vi "rem_killOcc.vi"(0 "Host_Reference":refnum<class "HGF_Reference.lvclass">, 2 "timeout in ms (-1)":i32, 3 "ID":string, 5 "error in (no error)":errorcluster) -> (14 "dup Host_Reference":refnum<class "HGF_Reference.lvclass">, 16 "dup timeout in ms (-1)":i32, 19 "error out":errorcluster)   [LabVIEW 2009, in "MoAgSy.lvlib" / "MoAgSy_Host.lvclass"]
doc: "<B>public</B> VI removes kill occurence from referenced Host.\nOccurrence is specified by the Agents ID.\n\nF.Berck@gsi.de\nGSI Darmstadt 2009"
uses:
  MoAgSy_Host.lvclass
  HGF_BaseClasses/HGF_Reference/HGF_Reference.lvclass
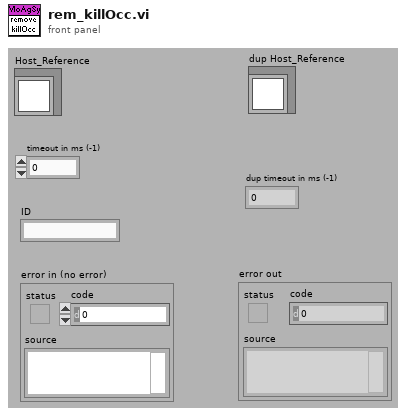
[diagram p1: front panel]
types:
  T1 = cluster{"killNotifier":refnum<notifier>, "Agent ID":string}[]
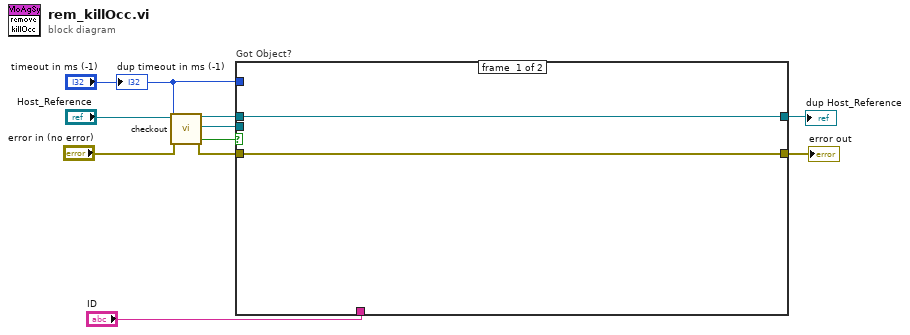
[diagram p0: block diagram]
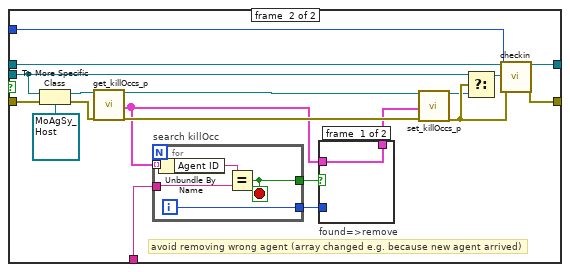
[diagram p2: hidden frame]
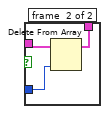
[diagram p3: hidden frame]
diagram:
  n1 = call "checkout.vi"("HGF_Reference"="Host_Reference", "timeout in ms (-1)"="timeout in ms (-1)", "error in (no error)"="error in (no error)") -> ("dup HGF_Reference"=w5:refnum<class "HGF_Reference.lvclass">, "Object"=w3:refnum<class>, "got object?"=w4:bool, "error out"=w2:errorcluster)  [unwired: 13 out]
  n2 = case "Got Object?" shown="True" w4 {
    tunnel: w3 -> [_ w25]
    tunnel: w5 -> [w12 w30]
    tunnel: [w12 w29] -> w8
    tunnel: "timeout in ms (-1)" -> [_ w28]
    tunnel: [w11 w27] -> w9
    tunnel: w2 -> [w11 w26]
    tunnel: "ID" -> [_ w17]
    frame #0 {
    }
    frame #1 {
      # "avoid removing wrong agent (array changed e.g. because new agent arrived)"
      n3 = To More Specific Class(target class=refnum<class "MoAgSy_Host.lvclass"> refnum ("MoAgSy.lvlib:MoAgSy_Host.lvclass"), reference=w25, error in=w26) -> (specific class reference=w23:refnum<class "MoAgSy_Host.lvclass">, error out=w22:errorcluster)
      n4 = call "get_killOccs_p.vi"("MoAgSy_Host"=w23, "error in (no error)"=w22) -> ("dup MoAgSy_Host"=w21:refnum<class "MoAgSy_Host.lvclass">, "Kill Occs"=w14:T1, "error out"=w20:errorcluster)  [unwired: 15 out]
      n5 = for "search killOcc" {
        tunnel: w14 -> [w40] mode=indexing
        tunnel: w17 -> [w38]
        tunnel: [w37] -> w16
        tunnel: [w36] -> w15
        i -> [w36]
        stop <- w37 stop-if-true
        n6 = Unbundle By Name(w40) -> ("Agent ID"=w39:string)
        n7 = Equal?(x=w39, y=w38) -> (x = y?=w37:bool)
      }
      n8 = case "found=>remove" shown="True" w16 {
        tunnel: w15 -> [_ w34]
        tunnel: w14 -> [w32 w35]
        tunnel: [w32 w33] -> w13
        frame #0 {
        }
        frame #1 {
          n9 = Delete From Array(array=w35, index=w34) -> (array with subset deleted=w33:T1)  [unwired: 1 in, 1 out]
        }
      }
      n10 = call "set_killOccs_p.vi"("MoAgSy_Host"=w21, "Kill Occs"=w13, "error in (no error)"=w20) -> ("dup MoAgSy_Host"=w18:refnum<class "MoAgSy_Host.lvclass">, "error out"=w19:errorcluster)  [unwired: 1 in, 14 out]
      n11 = Select(t=w25, s=w19, f=w18) -> (s? t:f=w24:refnum<class>)
      n12 = call "checkin.vi"("HGF_Reference"=w30, "Object"=w24, "timeout /ms (-1)"=w28, "error in (no error)"=w19) -> ("dup HGF_Reference"=w29:refnum<class "HGF_Reference.lvclass">, "error out"=w27:errorcluster)  [unwired: 14 out]
    }
  }
  "dup Host_Reference" <- w8
  "error out" <- w9
  "dup timeout in ms (-1)" <- "timeout in ms (-1)"
